vi "Set Board HW Entry.vi"(8 "boardresource":T1, 9 "InstrumentHandle_board":u32, 10 "boardId":u32, 11 "hw_data in":T2) -> (2 "duplicated":bool, 3 "hw_data out":T2)   [LabVIEW 2020, in "AIM664LV.lvlib"]
uses:
  AIM664LV.lvlib
  _controls/hwEntry_data.ctl
  _controls/hwEntryBoardHandleMap.ctl
  _controls/hwEntryBoardResource.ctl
  _controls/hwEntryPortResource.ctl
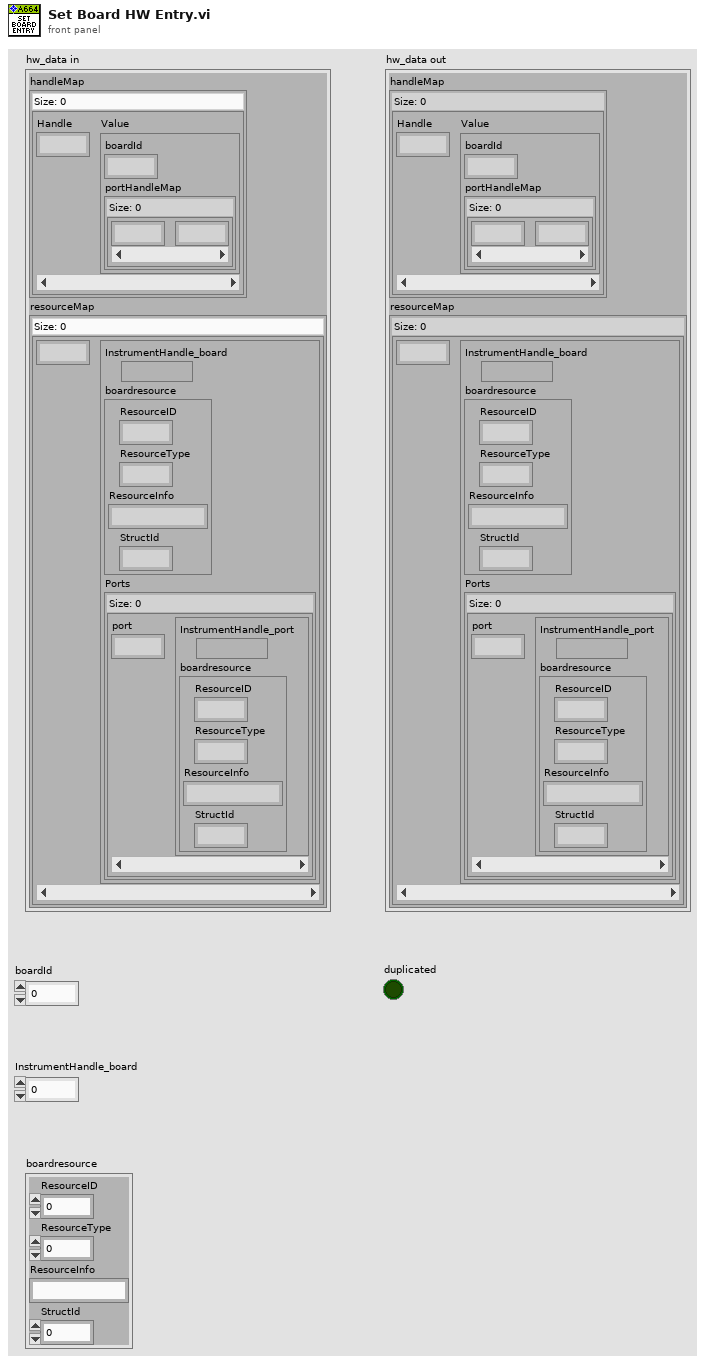
[diagram p1: front panel]
types:
  T1 = cluster{"ResourceID":u32, "ResourceType":u32, "ResourceInfo":string, "StructId":u32}
  T2 = typedef "AIM664LV.lvlib/hwEntry_data.ctl" = cluster{"handleMap":map{u32, T3}, "resourceMap":map{u32, T4}}
  T3 = typedef "AIM664LV.lvlib/hwEntryBoardHandleMap.ctl" = cluster{"boardId":u32, "portHandleMap":map{u32, u32}}
  T4 = typedef "AIM664LV.lvlib/hwEntryBoardResource.ctl" = cluster{"InstrumentHandle_board":u32, "boardresource":cluster{"ResourceID":u32, "ResourceType":u32, "ResourceInfo":string, "StructId":u32}, "Ports":map{u32, T5}}
  T5 = typedef "AIM664LV.lvlib/hwEntryPortResource.ctl" = cluster{"InstrumentHandle_port":u32, "boardresource":cluster{"ResourceID":u32, "ResourceType":u32, "ResourceInfo":string, "StructId":u32}}
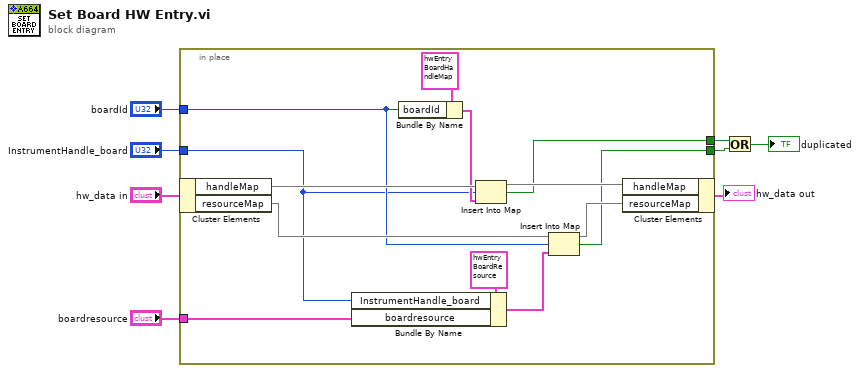
[diagram p0: block diagram]
diagram:
  n1 = in-place {
    in-place-border: "boardId" -> [w16]
    in-place-border: "InstrumentHandle_board" -> [w12]
    in-place-border: "boardresource" -> [w11]
    in-place-border: [w10] -> w3
    in-place-border: [w9] -> w2
    n2 = in-place-cluster #1("hw_data in") -> ("handleMap"=w20:map{u32, T3}, "resourceMap"=w17:map{u32, T4})
    n3 = Bundle By Name(cluster=T4 {"InstrumentHandle_board"=0, "boardresource"={"ResourceID"=0, "ResourceType"=0, "ResourceInfo"="", "StructId"=0}, "Ports"={}} ("value"), "InstrumentHandle_board"=w12, "boardresource"=w11) -> (w14:T4)
    n4 = Bundle By Name(cluster=T3 {"boardId"=0, "portHandleMap"={}}, "boardId"=w16) -> (w19:T3)
    n5 = Insert Into Map(map in=w20, key=w12, value=w19) -> (map out=w18:map{u32, T3}, key already included?=w10:bool)  [unwired: 1 out]
    n6 = Insert Into Map(map in=w17, key=w16, value=w14) -> (map out=w13:map{u32, T4}, key already included?=w9:bool)  [unwired: 1 out]
    n7 = in-place-cluster #1("handleMap"=w18, "resourceMap"=w13) -> (→"hw_data out":T2)
  }
  n8 = Or(x=w3, y=w2) -> (x .or. y?=→"duplicated":bool)
